vi "IMAQ balance energy.vi"(10 "Target Image":T1, 11 "Base Image":T1) -> (3 "Normalized Target":T1(plugin-control))   [LabVIEW 2012, in "LightPipes.lvlib"]
uses:
  LightPipes.lvlib
  <vilib>/vision/Image Controls.llb/IMAQ Image.ctl
panel:
  out "Ratio":dbl
  out "Target":u32
  out "Base":u32
  out "Normalized":u32
  # "1. Normalize Target.\n\n2. Scale Target's energy to Base's."
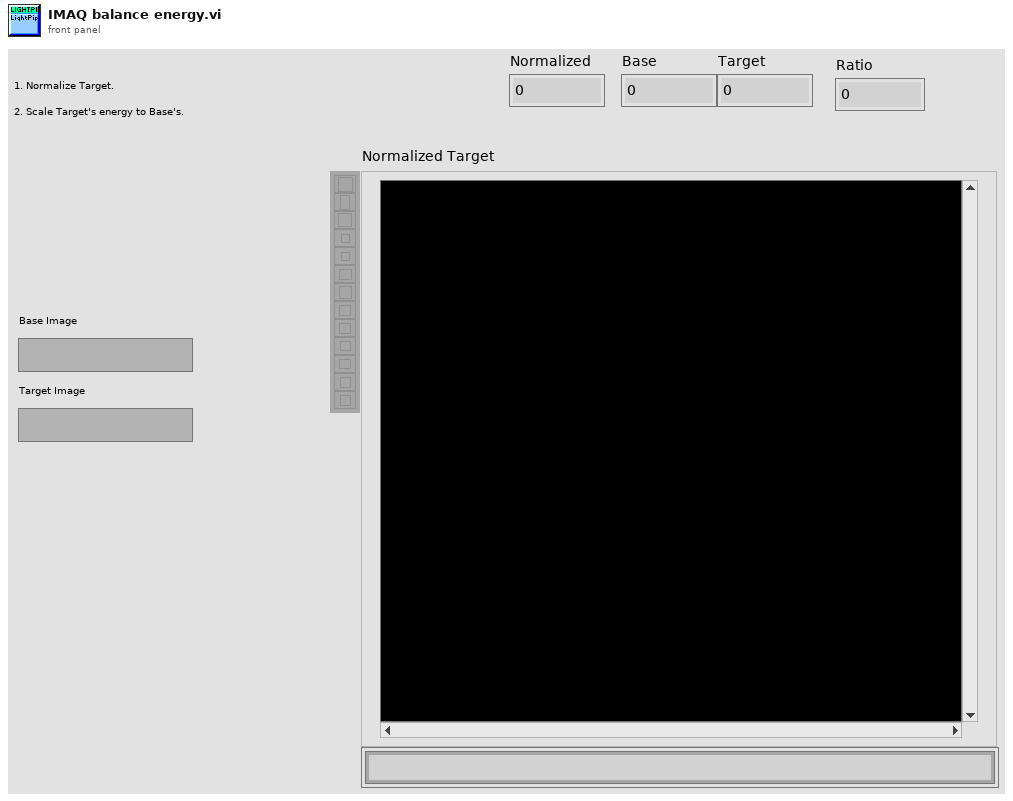
[diagram p1: front panel]
types:
  T1 = typedef "IMAQ Image.ctl" = refnum<image>
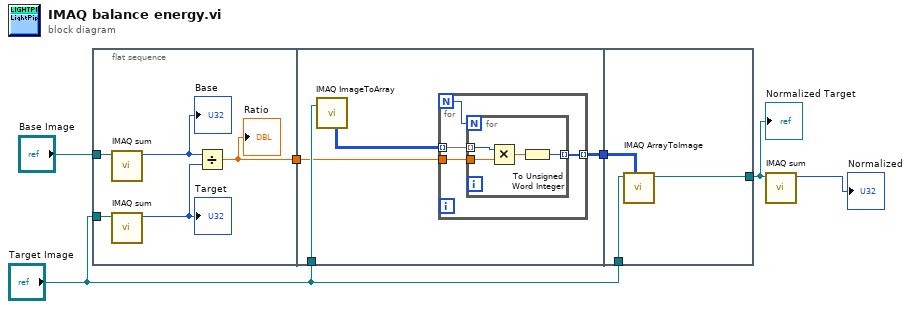
[diagram p0: block diagram]
diagram:
  n1 = flat-sequence {
    tunnel: "Base Image" -> [w11]
    tunnel: "Target Image" -> [w10]
    tunnel: [w7] -> w1
    tunnel: [w15] -> w5
    tunnel: "Target Image" -> [w14]
    tunnel: w1 -> [w12]
    tunnel: w5 -> [w24]
    tunnel: "Target Image" -> [w26]
    tunnel: [w25] -> w2
    frame #0 {
      n2 = call "IMAQ sum.vi"("Image"=w11) -> ("Sum"=w9:u32)  [unwired: 10 in]
      "Base" <- w9
      n3 = call "IMAQ sum.vi"("Image"=w10) -> ("Sum"=w8:u32)  [unwired: 10 in]
      "Target" <- w8
      n4 = Divide(x=w9, y=w8) -> (x/y=w7:dbl)
      "Ratio" <- w7
    }
    frame #1 {
      n5 = call "IMAQ ImageToArray"("Image"=w14) -> ("Image Pixels (U16)"=w13:u16[][])  [unwired: 3 in, 4 out]
      n6 = for {
        N -> [w19]
        tunnel: w13 -> [w18] mode=indexing
        tunnel: [w17] -> w15 mode=indexing
        tunnel: w12 -> [w16]
        n7 = for {
          N: w19 -> [_]
          tunnel: w18 -> [w20] mode=indexing
          tunnel: [w22] -> w17 mode=indexing
          tunnel: w16 -> [w21]
          n8 = Multiply(x=w20, y=w21) -> (x*y=w23:dbl)
          n9 = To Unsigned Word Integer(number=w23) -> (unsigned 16bit integer=w22:u16)
        }
      }
    }
    frame #2 {
      n10 = call "IMAQ ArrayToImage"("Image Pixels (U16)"=w24, "Image"=w26) -> ("Image Out"=w25:T1)  [unwired: 8 in, 1 out]
    }
  }
  n11 = call "IMAQ sum.vi"("Image"=w2) -> ("Sum"=→"Normalized":u32)  [unwired: 10 in]
  "Normalized Target" <- w2
